vi "ATE_Switches.vi"(8 "error in":errorcluster, 11 "ATE Switches":T2) -> (0 "Switch Errors":errorcluster, 3 "ATE Switch Status":T1={"Reversing Switch "=TRUE, "IO Switch #1"=TRUE, "IO Switch #2"=TRUE, "Signal Out"=TRUE, "Signal Source"=TRUE, "Power Meter"=TRUE, "Amp By Pass"=TRUE})   [LabVIEW 2012]
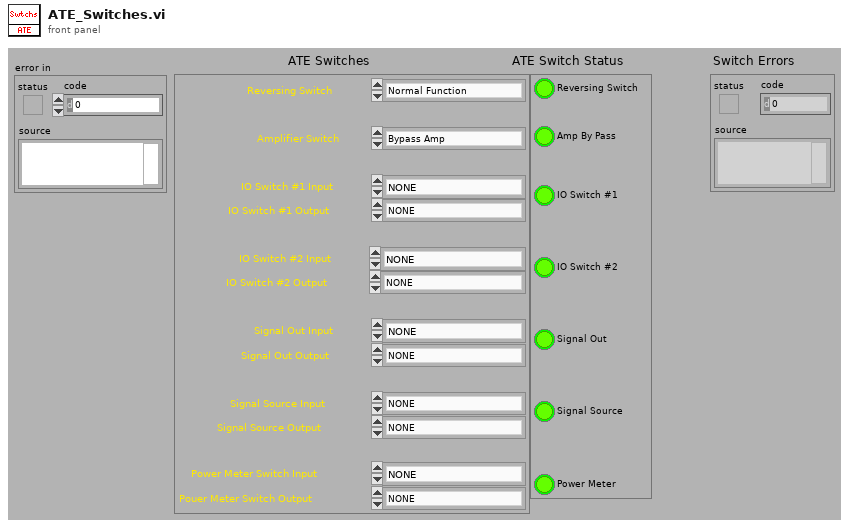
[diagram p1: front panel]
types:
  T1 = cluster{"Reversing Switch ":bool, "IO Switch #1":bool, "IO Switch #2":bool, "Signal Out":bool, "Signal Source":bool, "Power Meter":bool, "Amp By Pass":bool}
  T2 = cluster{"Reversing Switch":enum16{"Normal Function", "Reversing Function"}, "IO Switch #1 Input":enum16{"NONE", "AHR (J2)", "Splitter", "Signal Out Switch (S3)", "Reversing Switch"}, "IO Switch #1 Output":enum16{"NONE", "AHR (J2)", "Delay Device (S4)", "Power Meter Switch (S5)", "Reversing Switch"}, "IO Switch #2 Input":enum16{"NONE", "AVR (J3)", "Splitter", "Signal Out Switch (S3)", " 2W Term (TM1)", "Reversing Switch"}, "IO Switch #2 Output":enum16{"NONE", "AVR (J3)", "Signal Out Switch (S3)", "Power Meter Switch (S5)", "Reversing Switch", "2W Term (TM1)"}, "Signal Out Input":enum16{"NONE", "Amp Bypass Switch (S6)", "IO Switch #1 (S1)", "IO Switch #2 (S2)", "2W Term (TM3)"}, "Signal Out Output":enum16{"NONE", "2 Watt Term (TM3)", "Splitter", "Power Meter Switch (S5)"}, "Signal Source Input":enum16{"NONE", "Delay Device", "Signal Generator (J7)", "Inside Noise Box NF (J5)", "2W Term (TM3)"}, "Signal Source Output":enum16{"NONE", "Amp Bypass Switch", "Test Pulse Generator", "Power Meter Switch (S5)"}, "Power Meter Switch Input":enum16{"NONE", "IO Switch #1 (S1)", "Signal Source Switch (S4)", "Signal Out Switch (S3)", "IO Switch #2 (S2)", "TXH-TXV Switch (J8)"}, "Pouer Meter Switch Output":enum16{"NONE", "Power Meter (J6)"}, "Amplifier Switch":enum16{"Bypass Amp", "Include Amp"}}
  T3 = enum16{"NONE", "AHR (J2)", "Splitter", "Signal Out Switch (S3)", "Reversing Switch"}
  T4 = enum16{"NONE", "AHR (J2)", "Delay Device (S4)", "Power Meter Switch (S5)", "Reversing Switch"}
  T5 = enum16{"NONE", "AVR (J3)", "Splitter", "Signal Out Switch (S3)", " 2W Term (TM1)", "Reversing Switch"}
  T6 = enum16{"NONE", "AVR (J3)", "Signal Out Switch (S3)", "Power Meter Switch (S5)", "Reversing Switch", "2W Term (TM1)"}
  T7 = enum16{"NONE", "Amp Bypass Switch (S6)", "IO Switch #1 (S1)", "IO Switch #2 (S2)", "2W Term (TM3)"}
  T8 = enum16{"NONE", "2 Watt Term (TM3)", "Splitter", "Power Meter Switch (S5)"}
  T9 = enum16{"NONE", "Delay Device", "Signal Generator (J7)", "Inside Noise Box NF (J5)", "2W Term (TM3)"}
  T10 = enum16{"NONE", "Amp Bypass Switch", "Test Pulse Generator", "Power Meter Switch (S5)"}
  T11 = enum16{"NONE", "IO Switch #1 (S1)", "Signal Source Switch (S4)", "Signal Out Switch (S3)", "IO Switch #2 (S2)", "TXH-TXV Switch (J8)"}
  T12 = cluster{"Verfied":bool, "Verfied":bool, "Verfied":bool, "Verfied":bool, "Verfied":bool, "Verfied":bool, "Verfied":bool}
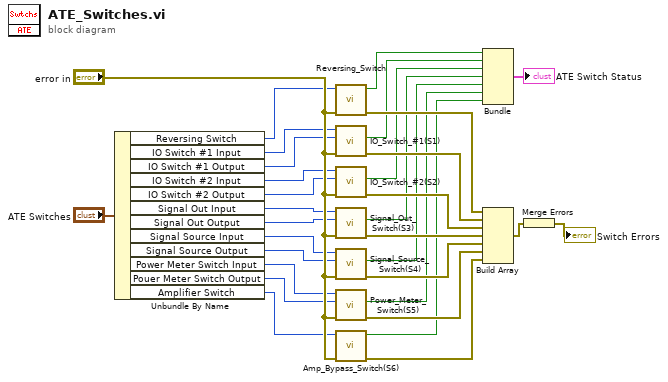
[diagram p0: block diagram]
diagram:
  n1 = Unbundle By Name("ATE Switches") -> ("Reversing Switch"=w20:enum16{"Normal Function", "Reversing Function"}, "IO Switch #1 Input"=w17:T3, "IO Switch #1 Output"=w11:T4, "IO Switch #2 Input"=w12:T5, "IO Switch #2 Output"=w13:T6, "Signal Out Input"=w14:T7, "Signal Out Output"=w15:T8, "Signal Source Input"=w1:T9, "Signal Source Output"=w2:T10, "Power Meter Switch Input"=w16:T11, "Pouer Meter Switch Output"=w18:enum16{"NONE", "Power Meter (J6)"}, "Amplifier Switch"=w19:enum16{"Bypass Amp", "Include Amp"})
  n2 = call "Reversing_Switch.vi"("error in"="error in", "Reversing Switch Function"=w20) -> ("error out"=w22:errorcluster, "Verfied"=w9:bool)  [unwired: 8 in]
  n3 = call "IO_Switch_#1(S1).vi"("error in"="error in", "Output"=w11, "Input"=w17) -> ("error out"=w23:errorcluster, "Verfied"=w8:bool)  [unwired: 6 in, 1 out]
  n4 = call "IO_Switch_#2(S2).vi"("error in"="error in", "Output"=w13, "Input"=w12) -> ("error out"=w24:errorcluster, "Verfied"=w7:bool)  [unwired: 6 in, 1 out]
  n5 = call "Signal_Out_Switch(S3).vi"("error in"="error in", "Output"=w15, "Input"=w14) -> ("error out"=w26:errorcluster, "Verfied"=w6:bool)  [unwired: 6 in, 1 out]
  n6 = call "Signal_Source_Switch(S4).vi"("error in"="error in", "Output"=w2, "Input"=w1) -> ("error out"=w27:errorcluster, "Verfied"=w5:bool)  [unwired: 6 in, 1 out]
  n7 = call "Power_Meter_Switch(S5).vi"("error in"="error in", "Output"=w18, "Input"=w16) -> ("error out"=w28:errorcluster, "Verfied"=w4:bool)  [unwired: 6 in, 1 out]
  n8 = call "Amp_Bypass_Switch(S6).vi"("error in"="error in", "AMP Function"=w19) -> ("error out"=w29:errorcluster, "Verfied"=w3:bool)  [unwired: 8 in]
  n9 = Bundle("Verfied"=w9, "Verfied"=w8, "Verfied"=w7, "Verfied"=w6, "Verfied"=w5, "Verfied"=w4, "Verfied"=w3) -> (→"ATE Switch Status":T12)  [unwired: 1 in]
  n10 = Build Array(w22, w23, w24, w26, w27, w28, w29) -> (w25:errorcluster[])
  n11 = Merge Errors(w25) -> (→"Switch Errors":errorcluster)
